vi "kolo_subvi.vi"() -> (3 "XY Graph":cluster{"X":dbl, "Y":dbl}[](graph))   [LabVIEW 2012]
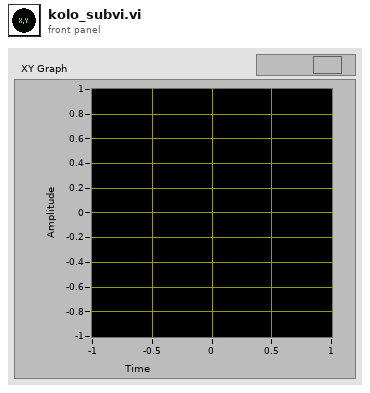
[diagram p1: front panel]
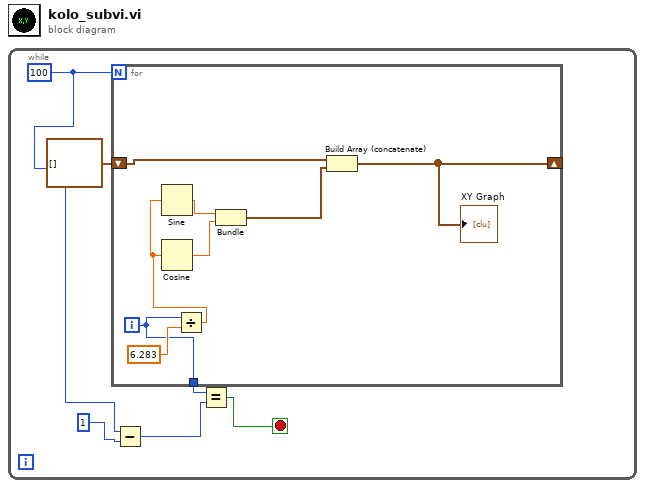
[diagram p0: block diagram]
diagram:
  n1 = while {
    stop <- w4 stop-if-true
    w2 = 100
    n2 = for {
      N: w2 -> [_]
      shift-right: [w8] -> _
      shift-left: cluster{dbl, dbl}[] [] -> [w13]
      tunnel: [w7] -> w5
      i -> [w7]
      n3 = Divide(x=w7, y=6.283) -> (x/y=w9:dbl)
      n4 = Sine(x=w9) -> (sin(x)=w11:dbl)
      n5 = Cosine(x=w9) -> (cos(x)=w10:dbl)
      n6 = Bundle(w11, w10) -> (w14:cluster{dbl, dbl})  [unwired: 1 in]
      n7 = Build Array (concatenate)(w13, w14) -> (w8:cluster{dbl, dbl}[])
      "XY Graph" <- w8
    }
    n8 = Subtract(x=w2, y=1) -> (x-y=w3:i32)
    n9 = Equal?(x=w5, y=w3) -> (x = y?=w4:bool)
  }
